vi "fft_wind_tester.vi"() -> ()   [LabVIEW 2021]
uses:
  <vilib>/measure/NI_MAPro.lvlib
  <vilib>/measure/maspectr.llb/FFT Power Spectrum and PSD for 1 Chan (CDB).vi
panel:
  out "Array":T1(array[cluster])
  out "cleanPSD":cluster{"f0":dbl, "df":dbl, "magnitude":dbl[]}(graph)
  out "fft":dbl[](graph)
  out "Array 2":i32[](array[numeric])
  out "F":i32[](graph)
  out "length":u16[](graph)
  out "amp":dbl[](graph)
  in  "amplitude bar":fxp<+,64,63>
  in  "#sampels":i32
  in  "amp":dbl
types:
  T1 = cluster{"PW":u16, "f":i32, "magnitude":fxp<+,32,31>}[]
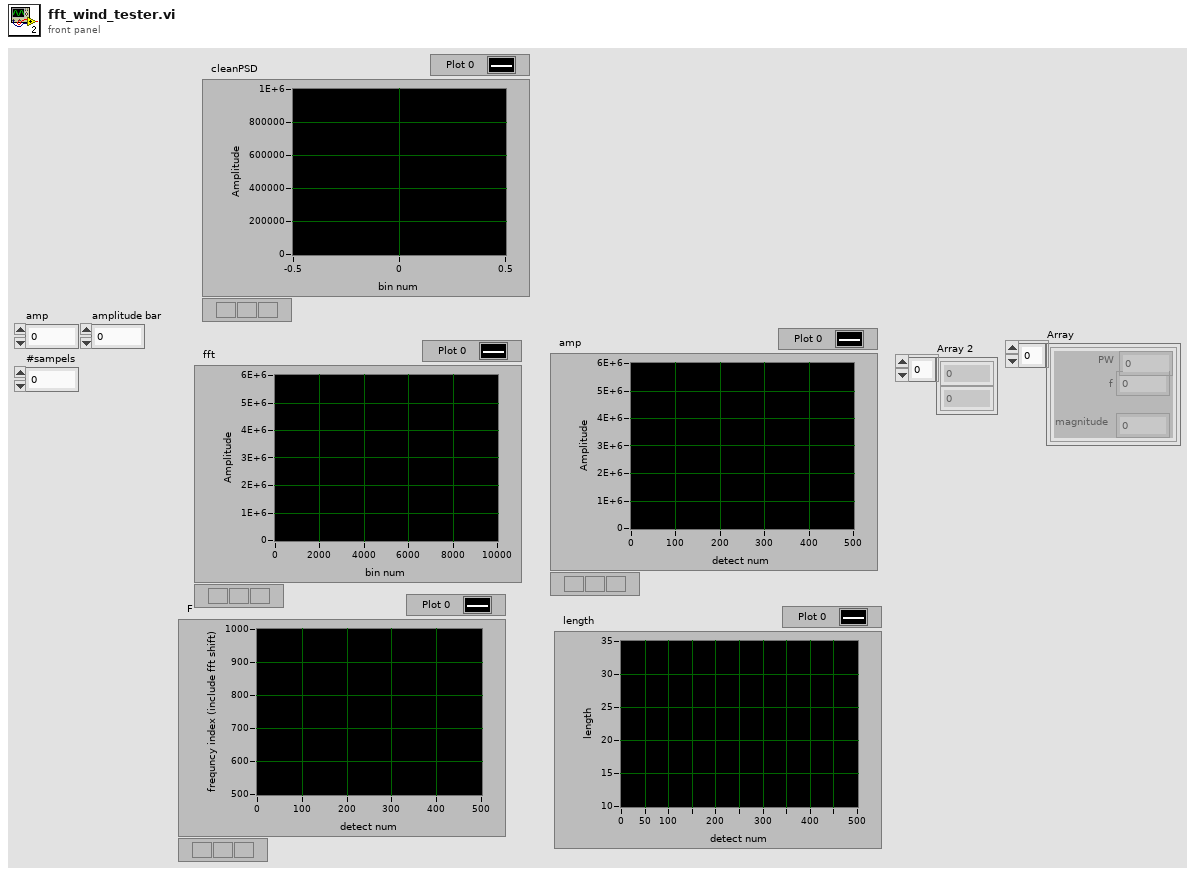
[diagram p1: front panel]
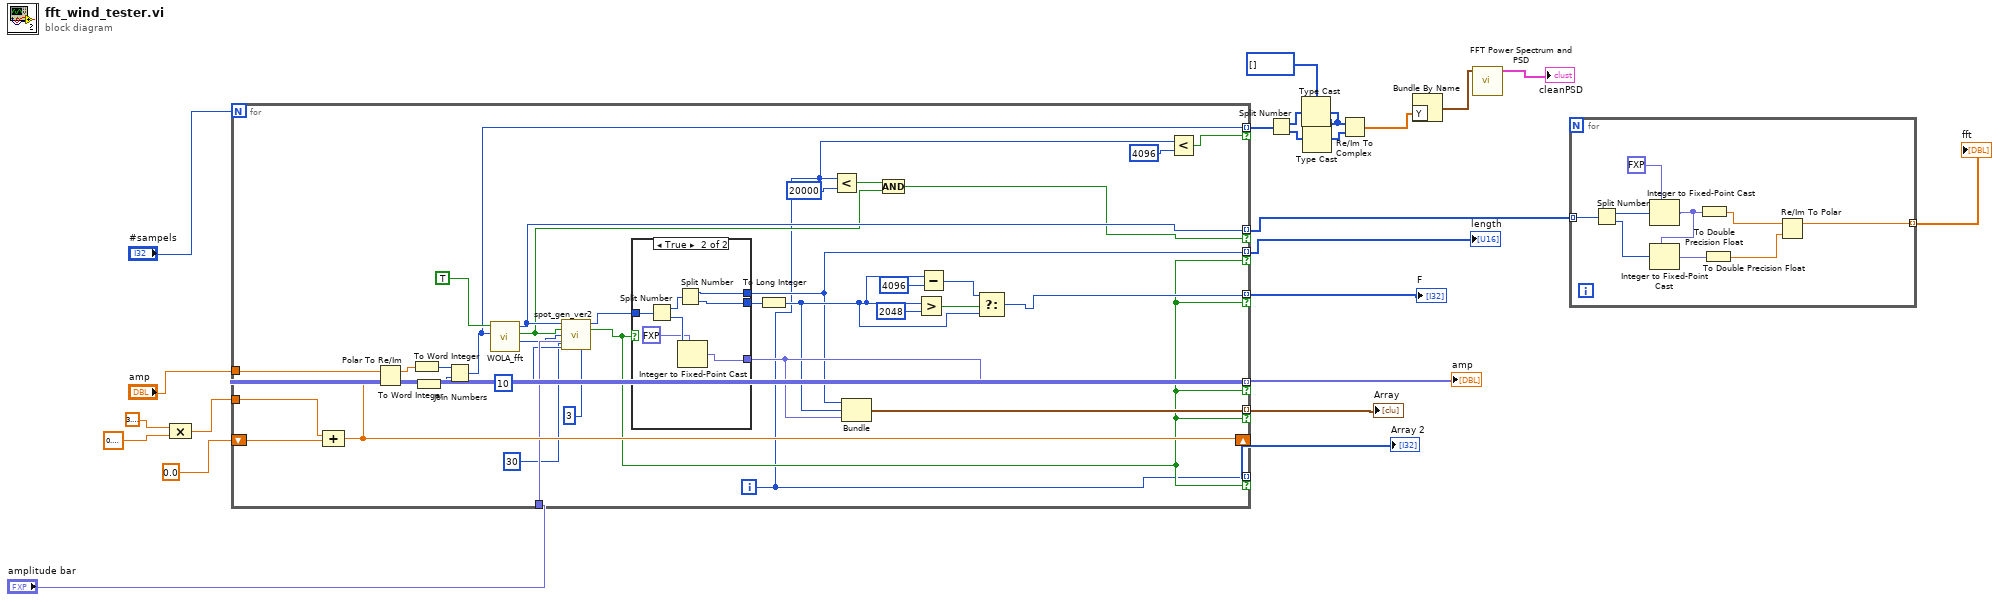
[diagram p0: block diagram]
diagram:
  n1 = Compound Arithmetic op=MULTIPLY(sgl 3.1415927, sgl 0.4 ("value")) -> (w20:sgl)
  n2 = for {
    N: "#sampels" -> [_]
    shift-right: [w55] -> _
    shift-left: 0.0 -> [w57]
    tunnel: w20 -> [w56]
    tunnel: "amp" -> [w54]
    tunnel: "amplitude bar" -> [w48]
    tunnel: [w33] -> w11 mode=indexing if=w30
    tunnel: [w38] -> w15 mode=indexing if=w35
    tunnel: [w44] -> w16 mode=indexing if=w35
    tunnel: [w43] -> w1 mode=indexing if=w35
    tunnel: [w24] -> w14 mode=indexing if=w35
    tunnel: [w34] -> w12 mode=indexing if=w35
    tunnel: [w27] -> w8 mode=indexing if=w25
    i -> [w24]
    n3 = Compound Arithmetic op=ADD(w56, w57) -> (w55:dbl)
    n4 = Polar To Re/Im(2:w55, 3:w54) -> (0:w52:dbl, 1:w53:dbl)
    n5 = To Word Integer(number=w53) -> (16bit integer=w51:i16)
    n6 = To Word Integer(number=w52) -> (16bit integer=w50:i16)
    n7 = Join Numbers(hi=w51, lo=w50) -> ((hi.lo)=w27:u32)
    n8 = call "WOLA_fft.vi"("data in"=w27, "input valid"=TRUE) -> ("data index"=w32:u16, "output valid"=w31:bool, "fft_output"=w33:u64)  [unwired: 6 in, 1 out]
    n9 = call "spot_gen_ver2.vi"("FFT_output"=w33, "input valid"=w31, "data index 2"=w32, "amplitude bar"=w48, "min PW"=u16 10, "max PW 2"=u16 30, "max gap"=u8 3) -> ("PDW"=w49:u64, "output valid"=w35:bool)  [unwired: 6 in, 1 out]
    n10 = case shown="True" w35 {
      tunnel: w49 -> [_ w62]
      tunnel: [_ w61] -> w37
      tunnel: [_ w60] -> w44
      tunnel: [_ w59] -> w34
      frame False {
      }
      frame True {
        n11 = Split Number(x=w62) -> (hi(x)=w65:u32, lo(x)=w64:u32)
        n12 = Split Number(x=w65) -> (hi(x)=w59:u16, lo(x)=w61:u16)
        n13 = Integer to Fixed-Point Cast(fixed-point type=fxp<+,32,31> 0.0 ("magnitude"), integer=w64) -> (fixed-point=w60:fxp<+,32,31>)
      }
    }
    n14 = To Long Integer(number=w37) -> (32bit integer=w36:i32)
    n15 = Less?(x=w24, y=20000) -> (x < y?=w29:bool)
    n16 = Bundle(w34, w36, "magnitude"=w44) -> (w43:cluster{u16, i32, "magnitude":fxp<+,32,31>})  [unwired: 1 in]
    n17 = And(x=w29, y=w31) -> (x .and. y?=w30:bool)
    n18 = Greater?(x=w36, y=u16 2048) -> (0:w41:bool)
    n19 = Subtract(x=w36, y=u16 4096) -> (x-y=w39:i32)
    n20 = Select(t=w39, s=w41, f=w36) -> (s? t:f=w38:i32)
    n21 = Less?(x=w24, y=4096) -> (x < y?=w25:bool)
  }
  "length" <- w12
  "F" <- w15
  "amp" <- w16
  "Array 2" <- w14
  "Array" <- w1
  n22 = Split Number(x=w8) -> (hi(x)=w7:u16[], lo(x)=w5:u16[])
  n23 = Type Cast(type=i16[] [] ("hi(x)"), x=w7) -> (*(type *) &x=w4:i16[])
  n24 = Type Cast(type=w4, x=w5) -> (*(type *) &x=w3:i16[])
  n25 = Re/Im To Complex(1:w3, 2:w4) -> (0:w2:cdb[])
  n26 = Bundle By Name("Y"=w2) -> (w9:waveform(cdb))  [unwired: 1 in]
  n27 = call-poly <vilib>:"FFT Power Spectrum and PSD.vi"("time signal"=w9) -> ("Power Spectrum / PSD"=→"cleanPSD":cluster{"f0":dbl, "df":dbl, "magnitude":dbl[]})  [unwired: 7 in, 3 out]
  n28 = for {
    tunnel: [w67] -> w13 mode=indexing
    tunnel: w11 -> [w66] mode=indexing
    n29 = Split Number(x=w66) -> (hi(x)=w73:u32, lo(x)=w72:u32)
    n30 = Integer to Fixed-Point Cast(fixed-point type=fxp<+/-,32,31> 0.0 ("I"), integer=w73) -> (fixed-point=w70:fxp<+/-,32,31>)
    n31 = Integer to Fixed-Point Cast(fixed-point type=w70, integer=w72) -> (fixed-point=w71:fxp<+/-,32,31>)
    n32 = To Double Precision Float(number=w70) -> (double precision float=w69:dbl)
    n33 = To Double Precision Float(number=w71) -> (double precision float=w68:dbl)
    n34 = Re/Im To Polar(2:w68, 3:w69) -> (1:w67:dbl)  [unwired: 1 out]
  }
  "fft" <- w13
